vi "Vision Server Remove Vision Update.vi"(1 "Vision Update":T2, 2 "Vision Server":T1) -> (0 "Vision Server":T1)   [LabVIEW 2016]
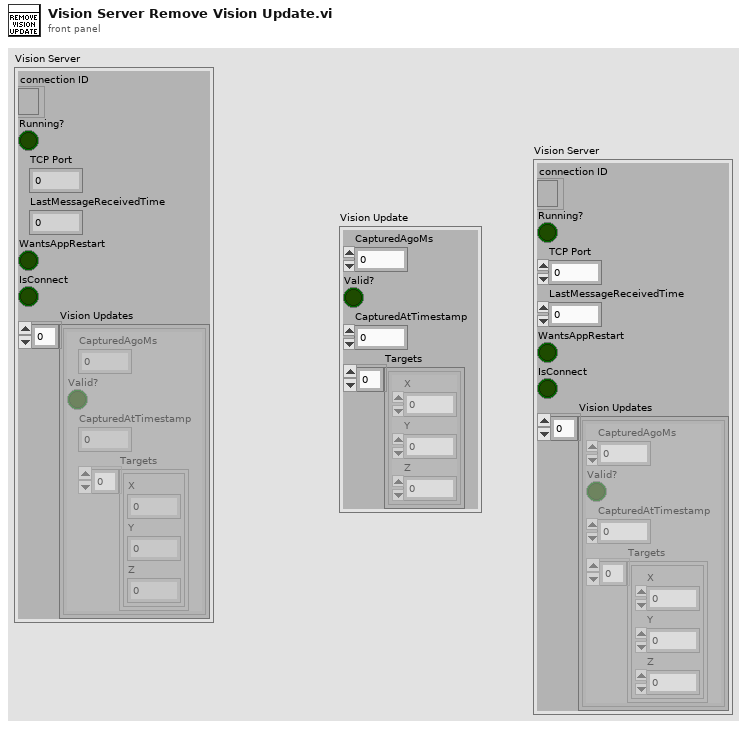
[diagram p1: front panel]
types:
  T1 = cluster{"connection ID":refnum<k5>, "Running?":bool, "TCP Port":u16, "LastMessageReceivedTime":dbl, "WantsAppRestart":bool, "IsConnect":bool, "Vision Updates":cluster{"CapturedAgoMs":i32, "Valid?":bool, "CapturedAtTimestamp":dbl, "Targets":cluster{"X":dbl, "Y":dbl, "Z":dbl}[]}[]}
  T2 = cluster{"CapturedAgoMs":i32, "Valid?":bool, "CapturedAtTimestamp":dbl, "Targets":cluster{"X":dbl, "Y":dbl, "Z":dbl}[]}
  T3 = cluster{"CapturedAgoMs":i32, "Valid?":bool, "CapturedAtTimestamp":dbl, "Targets":cluster{"X":dbl, "Y":dbl, "Z":dbl}[]}[]
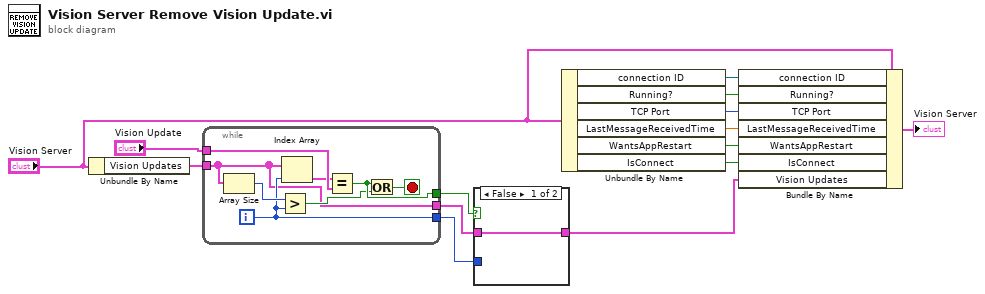
[diagram p0: block diagram]
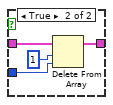
[diagram p2: hidden frame]
diagram:
  n1 = Unbundle By Name("Vision Server") -> ("Vision Updates"=w14:T3)
  n2 = while {
    tunnel: w14 -> [w15]
    tunnel: "Vision Update" -> [w22]
    tunnel: [w16] -> w10
    tunnel: [w20] -> w12
    tunnel: [w15] -> w11
    i -> [w16]
    stop <- w19 stop-if-true
    n3 = Array Size(array=w15) -> (size(s)=w17:i32)
    n4 = Greater?(x=w17, y=w16) -> (0:w18:bool)
    n5 = Index Array(array=w15, index=w16) -> (element=w21:T2)
    n6 = Equal?(x=w21, y=w22) -> (x = y?=w20:bool)
    n7 = Or(x=w20, y=w18) -> (x .or. y?=w19:bool)
  }
  n8 = case shown="False" w12 {
    tunnel: w11 -> [w23 w27]
    tunnel: w10 -> [_ w25]
    tunnel: [w23 w24] -> w3
    frame False {
    }
    frame True {
      n9 = Delete From Array(array=w27, length=1, index=w25) -> (array with subset deleted=w24:T3)  [unwired: 1 out]
    }
  }
  n10 = Unbundle By Name("Vision Server") -> ("connection ID"=w9:refnum<k5>, "Running?"=w8:bool, "TCP Port"=w7:u16, "LastMessageReceivedTime"=w6:dbl, "WantsAppRestart"=w5:bool, "IsConnect"=w4:bool)
  n11 = Bundle By Name(cluster="Vision Server", "connection ID"=w9, "Running?"=w8, "TCP Port"=w7, "LastMessageReceivedTime"=w6, "WantsAppRestart"=w5, "IsConnect"=w4, "Vision Updates"=w3) -> (→"Vision Server":T1)
